vi "az_to_rad_back.vi"(1 "az quantity":u8, 2 "az":u8) -> (0 "rad":dbl)   [LabVIEW 2015]
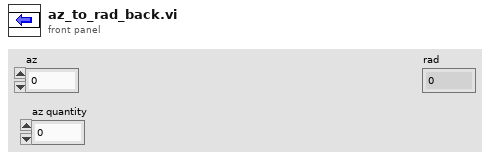
[diagram p1: front panel]
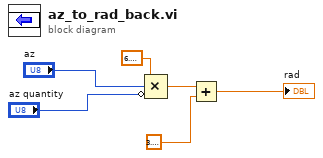
[diagram p0: block diagram]
diagram:
  n1 = Compound Arithmetic op=MULTIPLY(6.283185307179586, "az", invert "az quantity") -> (w4:dbl)
  n2 = Add(x=w4, y=3.141592653589793) -> (x+y=→"rad":dbl)
